vi "Pockels Cal-Initilise cal editor window.vi"(7 "Function":T1(ring), 8 "error in (no error)":errorcluster, 9 "Cal Wav listbox":refnum<vi>, 10 "Cal files listbox":refnum<vi>, 11 "XYGraph in":refnum<vi>) -> (0 "error out":errorcluster, 1 "SINGLE CAL SET / Pockels Cal table (inc. headers & info)":string[][](array[string]), 2 "All data loaded":string[][](array[string]), 3 "XYGraph out":refnum<vi>)   [LabVIEW 2013]
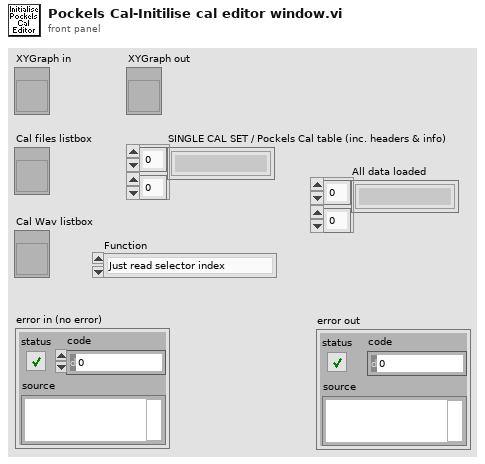
[diagram p1: front panel]
types:
  T1 = enum16{"Just read selector index", "remap to selected cal", "map to active cal"}
  T2 = enum16{"Set cursors dynamically", "Set cursors from file"}
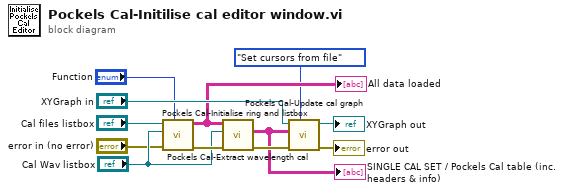
[diagram p0: block diagram]
diagram:
  n1 = call "Pockels Cal-Initialise ring and listbox.vi"("Function"="Function", "error in (no error)"="error in (no error)", "Cal Wav listbox"="Cal Wav listbox", "Cal files listbox"="Cal files listbox") -> ("error out"=w11:errorcluster, "All data loaded"=w5:string[][])  [unwired: 6 in]
  "All data loaded" <- w5
  n2 = call "Pockels Cal-Extract wavelength cal.vi"("error in (no error)"=w11, "Cal Wav listbox"="Cal Wav listbox", "All data loaded"=w5) -> ("error IO"=w7:errorcluster, "SINGLE CAL SET / Pockels Cal table (inc. headers & info)"=w6:string[][])  [unwired: 7 in]
  "SINGLE CAL SET / Pockels Cal table (inc. headers & info)" <- w6
  n3 = call "Pockels Cal-Update cal graph.vi"("Function"=T2."Set cursors from file", "error in (no error)"=w7, "Cal table"=w6, "XYGraph in"="XYGraph in") -> ("error out"=→"error out":errorcluster, "XYGraph"=→"XYGraph out":refnum<vi>)  [unwired: 6 in]
